vi "AdventCode_CleanUp.vi"(8 "Error In":errorcluster) -> (0 "Error Out":errorcluster)   [LabVIEW 2020, in "AdventCode.lvclass"]
uses:
  AdventCode.lvclass
  AdventCode.lvclass/AdventCode.ctl
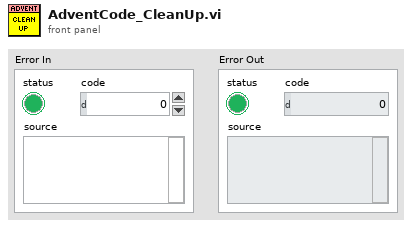
[diagram p1: front panel]
types:
  T1 = typedef "AdventCode.lvclass/ObjectAttributes.ctl" = cluster{"Year":i32, "Day":i32, "PuzzleData":string}
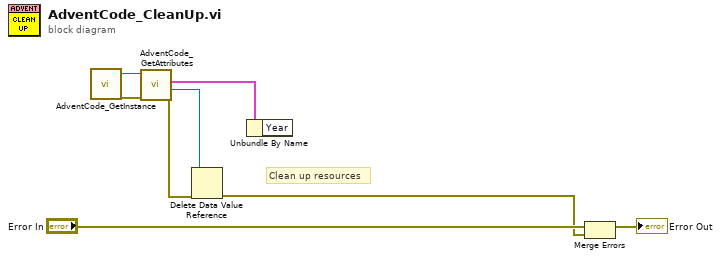
[diagram p0: block diagram]
diagram:
  # "Clean up resources"
  n1 = call "AdventCode_GetInstance.vi"() -> ("error out"=w6:errorcluster, "reference out"=w5:refnum<class "AdventCode.lvclass">)  [unwired: 7 in, 3 out]
  n2 = call "AdventCode_GetAttributes.vi"("error in (no error)"=w6, "reference in"=w5) -> ("error out"=w4:errorcluster, "DataRef"=w3:refnum<data-value>, "Data"=w7:T1)  [unwired: 6 in, 1 out]
  n3 = Delete Data Value Reference(data value reference=w3, error in=w4) -> (error out=w1:errorcluster)  [unwired: 1 out]
  n4 = Unbundle By Name(w7) -> ()  [unwired: 1 out]
  n5 = Merge Errors("Error In", w1) -> (→"Error Out":errorcluster)
